vi "OM_ToLabVIEW.vi"(8 "error in (no error)":errorcluster, 10 "DbRow":variant, 11 "syslogs in":refnum<class "syslogs.lvclass">) -> (0 "error out":errorcluster, 1 "found":bool, 3 "syslogs out":refnum<class "syslogs.lvclass">)   [LabVIEW 2020, in "ORM_Examples.lvlib" / "syslogs.lvclass"]
uses:
  syslogs.lvclass
  syslogs.lvclass/syslogs.ctl
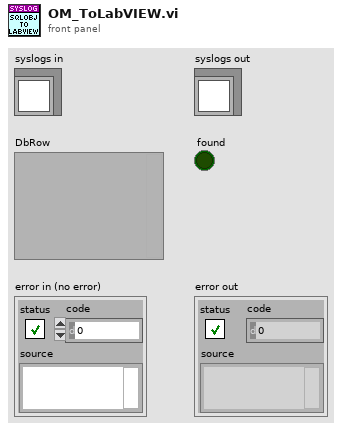
[diagram p1: front panel]
types:
  T1 = typedef "ORM_Examples.lvlib/syslogs.lvclass/type.ctl" = string
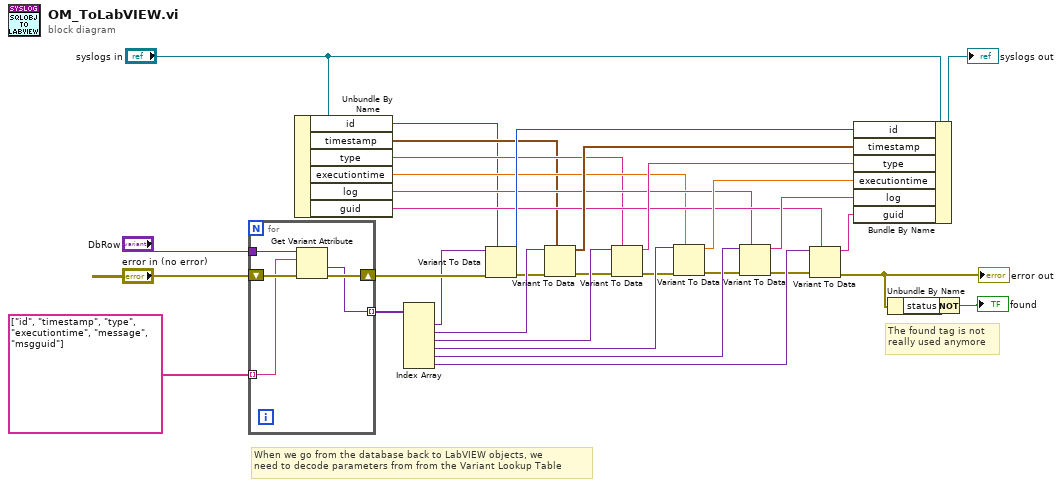
[diagram p0: block diagram]
diagram:
  # "The found tag is not \nreally used anymore"
  # "When we go from the database back to LabVIEW objects, we\nneed to decode parameters from from the Variant Lookup Table"
  n1 = for {
    shift-right: [w37] -> w29
    shift-left: "error in (no error)" -> [w38]
    tunnel: string[] ["id", "timestamp", "type", "executiontime", "message", "msgguid"] -> [w36] mode=indexing
    tunnel: "DbRow" -> [w35]
    tunnel: [w34] -> w15 mode=indexing
    n2 = Get Variant Attribute(Variant=w35, name=w36, error in=w38) -> (value=w34:variant, error out=w37:errorcluster)  [unwired: 1 in, 2 out]
  }
  n3 = Unbundle By Name("syslogs in") -> ("id"=w16:i32, "timestamp"=w17:timestamp, "type"=w18:T1, "executiontime"=w19:dbl, "log"=w20:string, "guid"=w21:string)
  n4 = Index Array(array=w15) -> (element #1=w14:variant, element #2=w13:variant, element #3=w12:variant, element #4=w11:variant, element #5=w10:variant, element #6=w9:variant)  [unwired: 6 in]
  n5 = Variant To Data(error in=w29, type=w16, Variant=w14) -> (data=w27:i32, error out=w8:errorcluster)
  n6 = Variant To Data(error in=w8, type=w17, Variant=w13) -> (data=w26:timestamp, error out=w7:errorcluster)
  n7 = Variant To Data(error in=w7, type=w18, Variant=w12) -> (data=w25:T1, error out=w6:errorcluster)
  n8 = Variant To Data(error in=w6, type=w19, Variant=w11) -> (data=w24:dbl, error out=w5:errorcluster)
  n9 = Variant To Data(error in=w5, type=w20, Variant=w10) -> (data=w23:string, error out=w4:errorcluster)
  n10 = Variant To Data(error in=w4, type=w21, Variant=w9) -> (data=w22:string, error out=w3:errorcluster)
  "error out" <- w3
  n11 = Bundle By Name(cluster="syslogs in", "id"=w27, "timestamp"=w26, "type"=w25, "executiontime"=w24, "log"=w23, "guid"=w22) -> (→"syslogs out":refnum<class "syslogs.lvclass">)
  n12 = Unbundle By Name(w3) -> ("status"=w2:bool)
  n13 = Not(x=w2) -> (.not. x?=→"found":bool)
